vi "Translation_GetXY.vi"(11 "In Translation":T1) -> (1 "Y":dbl, 3 "X":dbl)   [LabVIEW 2019, in "Trajectory_Library.lvlib"]
doc: "Returns the X and Ycomponents of the translation.\n\nParameters\n - IN Translation - This Translation data structure\n\nReturns:\n - X- The X component of the translation.\n - Y- The Y component of the translation."
uses:
  Trajectory_Library.lvlib
  TRANSLATION2D.ctl
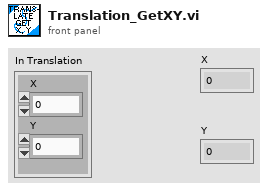
[diagram p1: front panel]
types:
  T1 = typedef "Trajectory_Library.lvlib/TRANSLATION2D.ctl" = cluster{"X":dbl, "Y":dbl}
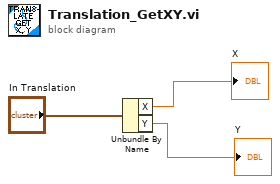
[diagram p0: block diagram]
diagram:
  n1 = Unbundle By Name("In Translation") -> ("X"=→"X":dbl, "Y"=→"Y":dbl)
